vi "Cancel Basic info.vi"(8 "error in (no error)":errorcluster caption="에러 입력(에러 없음)") -> (0 "error out":errorcluster caption="에러 출력", 2 "불리언":bool, 3 "교정환경":T1, 4 "item names":string[][](array[string]), 5 "교정정보":T2, 6 "교정절차 목록 MC List":i32, 7 "등록번호":string)   [LabVIEW 2020]
uses:
  Controls/Clst_Cal Info Global.ctl
  Controls/Clst_Atm Info Global.ctl
  Variables/Global_Cal Info.vi
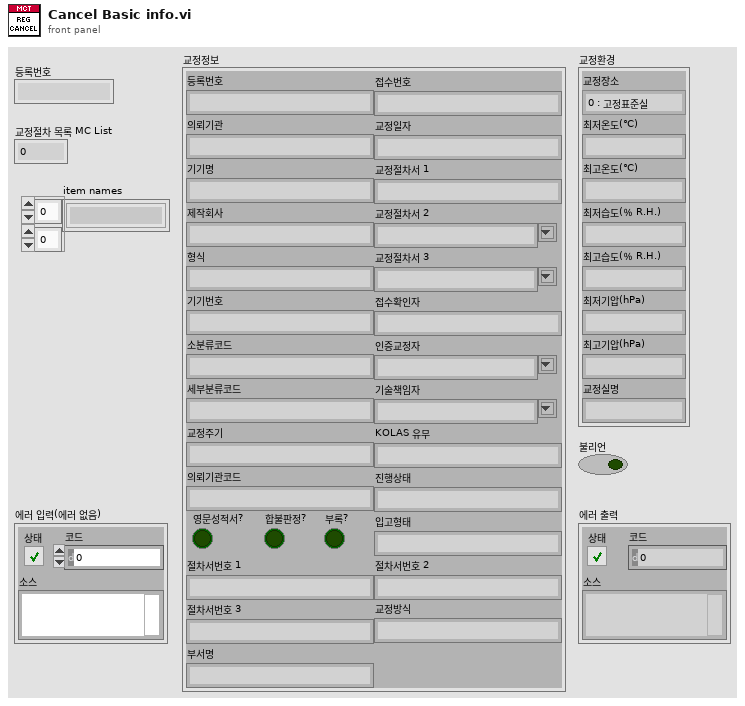
[diagram p1: front panel]
types:
  T1 = typedef "Clst_Atm Info Global.ctl" = cluster{"교정장소":enum16{"0 : 고정표준실", "1 : 현장교정"}, "최저온도(℃)":string, "최고온도(℃)":string, "최저습도(％ R.H.)":string, "최고습도(％ R.H.)":string, "최저기압(hPa)":string, "최고기압(hPa)":string, "교정실명":string}
  T2 = typedef "Clst_Cal Info Global.ctl" = cluster{"등록번호":string, "의뢰기관":string, "기기명":string, "제작회사":string, "형식":string, "기기번호":string, "소분류코드":string, "세부분류코드":string, "교정주기":string, "접수번호":string, "교정일자":string, "교정절차서 1":string, "교정절차서 2":string, "교정절차서 3":string, "접수확인자":string, "인증교정자":string, "기술책임자":string, "KOLAS 유무":string, "진행상태":string, "의뢰기관코드":string, "입고형태":string, "영문성적서?":bool, "합불판정?":bool, "부록?":bool, "절차서번호 1":string, "절차서번호 2":string, "절차서번호 3":string, "교정방식":string, "부서명":string}
  T3 = cluster{"세부분류코드":string, "형식":string, "옵션":string, "측정기명":string, "EXCEL파일명":string, "TEMP":string}
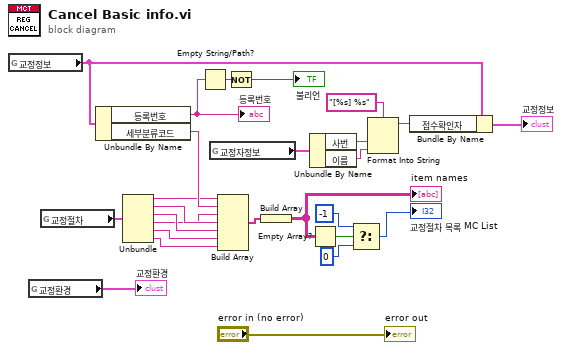
[diagram p0: block diagram]
diagram:
  n1 = global read "Global_Cal Info.vi" "교정정보"() -> (w18:T2)
  n2 = global read "Global_Cal Info.vi" "교정환경"() -> (→"교정환경":T1)
  n3 = global read "Global_Cal Info.vi" "교정절차"() -> (w5:T3)
  n4 = Unbundle By Name(w18) -> ("등록번호"=w23:string, "세부분류코드"=w19:string)
  "등록번호" <- w23
  n5 = Unbundle(w5) -> ("세부분류코드"=w6:string, "형식"=w21:string, "옵션"=w22:string, "측정기명"=w20:string, "EXCEL파일명"=w26:string, "TEMP"=w1:string)
  n6 = Empty String/Path?(string/path=w23) -> (empty?=w24:bool)
  n7 = global read "Global_Cal Info.vi" "교정자정보"() -> (w13:cluster{"사번":string, "이름":string, "자격":string})
  n8 = Build Array(w6, w19, w20, w21, w22, w26, w1) -> (w3:string[])
  n9 = Not(x=w24) -> (.not. x?=→"불리언":bool)
  n10 = Build Array(w3) -> (w7:string[][])
  "item names" <- w7
  n11 = Unbundle By Name(w13) -> ("사번"=w14:string, "이름"=w15:string)
  n12 = Empty Array?(array=w7) -> (empty?=w8:bool)
  n13 = Select(t=-1 ("교정절차 목록 MC List"), s=w8, f=0 ("교정절차 목록 MC List")) -> (s? t:f=→"교정절차 목록 MC List":i32)
  n14 = Format Into String(format string="[%s] %s" ("포맷 문자열"), w14, w15) -> (resulting string=w12:string)  [unwired: 2 in, 1 out]
  n15 = Bundle By Name(cluster=w18, "접수확인자"=w12) -> (→"교정정보":T2)
  "error out" <- "error in (no error)"
